vi "projector_image_to_camera_image_subvi.vi"(6 "Camera dot radius":i32, 7 "transformation_description":dbl[](array[numeric])=[1.0, 0.0, 1.0, 0.0, 0.0], 8 "error in (no error)":errorcluster, 9 "Converted Camera Image In":T1, 10 "Projector Image In":T1, 11 "Projector to Camera Calibration":T1) -> (0 "error out":errorcluster, 3 "Converted Camera Image Out":T1)   [LabVIEW 2019]
uses:
  <vilib>/vision/Image Controls.llb/IMAQ Image.ctl
  <vilib>/vision/NI_Vision_Development_Module.lvlib
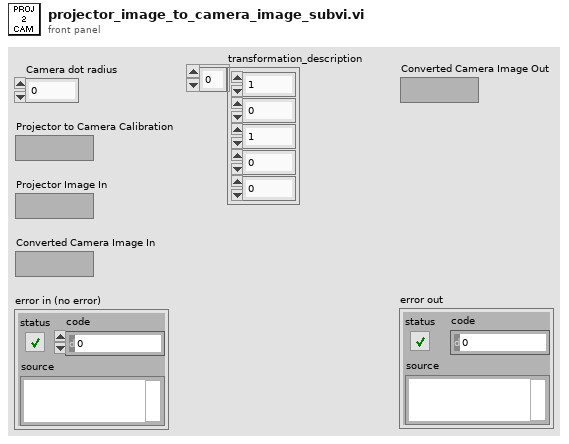
[diagram p1: front panel]
types:
  T1 = typedef "IMAQ Image.ctl" = refnum<image>
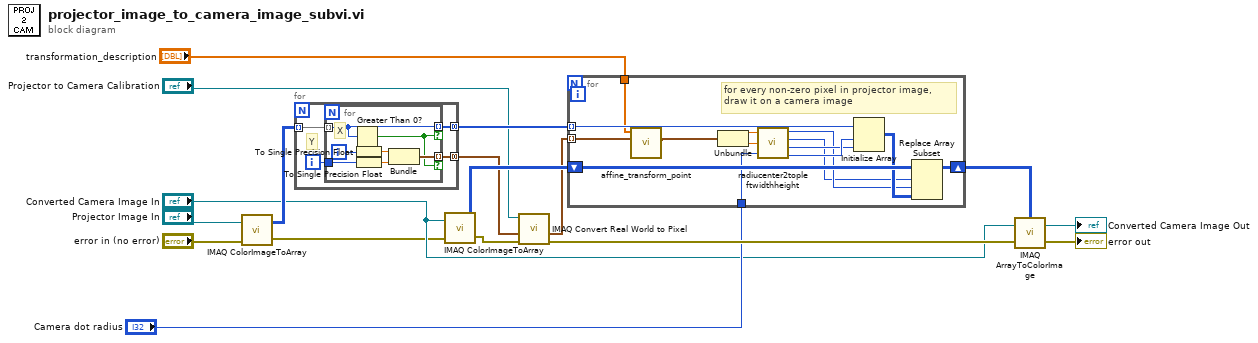
[diagram p0: block diagram]
diagram:
  n1 = call "IMAQ ColorImageToArray"("Image"="Projector Image In", "error in (no error)"="error in (no error)") -> ("Image Pixels (U32)"=w9:u32[][], "error out"=w2:errorcluster)  [unwired: 2 in, 1 out]
  n2 = for {
    tunnel: w9 -> [w21] mode=indexing
    tunnel: [w19] -> w5 mode=concatenating
    tunnel: [w18] -> w6 mode=concatenating
    i -> [w20]
    # "Y"
    n3 = for {
      tunnel: w21 -> [w22] mode=indexing
      tunnel: w20 -> [w27]
      tunnel: [w24] -> w18 mode=indexing if=w23
      tunnel: [w22] -> w19 mode=indexing if=w23
      i -> [w28]
      # "X"
      n4 = Greater Than 0?(x=w22) -> (x > 0?=w23:bool)
      n5 = To Single Precision Float(number=w28) -> (single precision float=w26:sgl)
      n6 = To Single Precision Float(number=w27) -> (single precision float=w25:sgl)
      n7 = Bundle(w26, w25) -> (w24:cluster{sgl, sgl})  [unwired: 1 in]
    }
  }
  n8 = call "IMAQ ColorImageToArray"("Image"="Converted Camera Image In", "error in (no error)"=w2) -> ("Image Pixels (U32)"=w11:u32[][], "error out"=w16:errorcluster)  [unwired: 2 in, 1 out]
  n9 = call "IMAQ Convert Real World to Pixel"("error in (no error)"=w16, "Array of Real World Coordinates"=w6, "Calibrated Image"="Projector to Camera Calibration") -> ("error out"=w17:errorcluster, "Array of Pixel Coordinates"=w7:cluster{"X":sgl, "Y":sgl}[])  [unwired: 3 in, 4 out]
  n10 = for {
    tunnel: w5 -> [w39] mode=indexing
    tunnel: w7 -> [w31] mode=indexing
    shift-right: [w37] -> w12
    shift-left: w11 -> [w40]
    tunnel: "Camera dot radius" -> [w36]
    tunnel: "transformation_description" -> [w29]
    # "for every non-zero pixel in projector image, \ndraw it on a camera image"
    n11 = call "affine_transform_point.vi"("Pixel Coordinates In"=w31, "transformation_description"=w29) -> ("Pixel Coordinates Out"=w30:cluster{"X":sgl, "Y":sgl})  [unwired: 9 in]
    n12 = Unbundle(w30) -> ("X"=w42:sgl, "Y"=w41:sgl)
    n13 = call "radiucenter2topleftwidthheight.vi"("Radius"=w36, "ycenter"=w41, "xcenter"=w42) -> ("Height"=w35:i32, "Width"=w34:i32, "Top"=w32:i32, "Left"=w33:i32)  [unwired: 2 in]
    n14 = Initialize Array(w39, w35, w34) -> (w38:u32[][])
    n15 = Replace Array Subset(array=w40, new element=w38, index (row)=w32, index (col)=w33) -> (w37:u32[][])
  }
  n16 = call "IMAQ ArrayToColorImage"("Image Pixels (U32)"=w12, "Image"="Converted Camera Image In", "error in (no error)"=w17) -> ("Image Out"=→"Converted Camera Image Out":T1, "error out"=→"error out":errorcluster)  [unwired: 2 in]
